vi "camara y sonido.vi"() -> ()   [LabVIEW 2010]
uses:
  <vilib>/sound2/lvsound2.llb/Sound Data Format.ctl
  <vilib>/addons/PixeLINK/Low Level Functions/CAMERA_FEATURES.llb/TDPU-CameraFeatures-PixelFormat.ctl
  <vilib>/sound2/lvsound2.llb/Sound Output Task ID.ctl
  <vilib>/vision/Image Controls.llb/IMAQ Image.ctl
panel:
  in  "Salto a Base":bool
  in  "Comienza Saltos":bool
  out "Estable":bool=TRUE
  out "Saltando":bool=TRUE
  in  "Path":path
  in  "Nombre Imagen":string="foto"
  in  "Numero Ultimo Experimento":i32
  in  "Parametros de Saltos":T1={"Numero de Saltos"=6, "Paso del Salto (Hz)"=100.0, "Tiempo de estabilizacion (s)"=1.0, "Frequencia de estabilizacion (Hz)"=2000.0, "Tiempo de rampa ON (s)"=5.0, "Tiempo de rampa OFF (s)"=1.0}
  in  "Calibrar Sonido":bool
  out "Archivo Actual":path
  out "Guardando Imagen":bool=TRUE
  in  "Compresion":u16(ring)=6 items=["DV Video Encoder", "LogMeIn Video Encoder", "MJPEG Compressor", "Cinepak Codec by Radius", "Intel IYUV codec", "Intel IYUV codec", "Microsoft RLE", "Microsoft Video 1"]
  in  "Nueva Linea?":bool
  in  "Grabar":bool
  in  "Video?":bool
  out "Archivo de texto":path
  out "Selected Path for AVI":path
  out "time (ms)":u32
  out "Contraste":dbl(graph)
  out "Todo Funciona?":bool
  out "Image":T2(plugin-control)
  in  "Tab Control":enum32{"Sound", "Camara"}(tab)
  in  "Sound Controls":T4={"device ID"=0, "sound format"={"sample rate (S/s)"=44000.0, "number of channels"=2, "bits per sample"=16}, "time (ms)"=200.0}
  in  "Sound?":bool
  in  "Frecuencia":dbl
  in  "Selector":u16(ring) items=["776002034"]
  in  "Streeam?":bool
  out "Camara Funciona?":bool
  out "Contraste":dbl
  in  "Camera Parameters":T6 {"Pixel Format" items=["PIXEL_FORMAT_MONO8", "PIXEL_FORMAT_MONO16", "PIXEL_FORMAT_YUV422", "PIXEL_FORMAT_BAYER8_GRBG", "PIXEL_FORMAT_BAYER16_GRBG", "PIXEL_FORMAT_RGB24", "PIXEL_FORMAT_RGB48", "PIXEL_FORMAT_BAYER8_RGGB", "PIXEL_FORMAT_BAYER8_GBRG ", "PIXEL_FORMAT_BAYER8_BGGR ", "PIXEL_FORMAT_BAYER16_RGGB ", "PIXEL_FORMAT_BAYER16_GBRG", "PIXEL_FORMAT_BAYER16_BGGR", "PIXEL_FORMAT_RGB32"]}
  in  "stop":bool
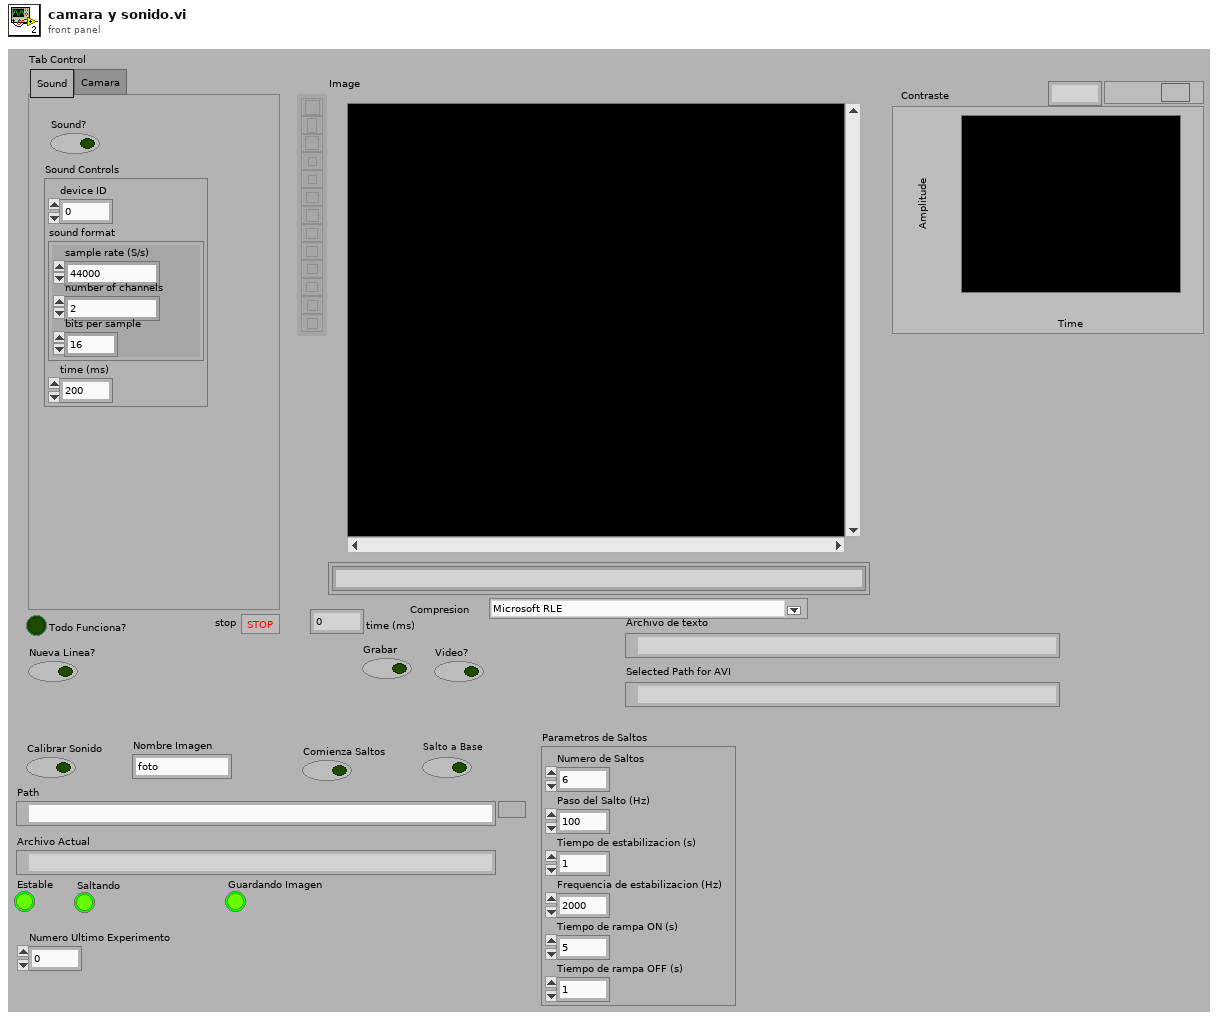
[diagram p1: front panel]
types:
  T1 = cluster{"Numero de Saltos":i32, "Paso del Salto (Hz)":dbl, "Tiempo de estabilizacion (s)":dbl, "Frequencia de estabilizacion (Hz)":dbl, "Tiempo de rampa ON (s)":dbl, "Tiempo de rampa OFF (s)":dbl}
  T2 = typedef "IMAQ Image.ctl" = refnum<image>
  T3 = typedef "Sound Data Format.ctl" = cluster{"sample rate (S/s)":dbl, "number of channels":i32, "bits per sample":i32}
  T4 = cluster{"device ID":u32, "sound format":T3, "time (ms)":dbl}
  T5 = typedef "TDPU-CameraFeatures-PixelFormat.ctl" = u16
  T6 = cluster{"Exposure Time (ms)":dbl, "Gain (dB)":dbl, "Saturation (%)":dbl, "Sharpness (%)":dbl, "Color Temperature":dbl, "ROI":cluster{"Top":i32, "Left":i32, "Width":i32, "Height":i32}, "White Balance Gain (dB)":cluster{"Red":dbl, "Green":dbl, "Blue":dbl}, "Gamma":dbl, "Pixel Format":T5, "FPS (frames/s)":i32}
  T7 = cluster{"hCamera":u32, "Error":errorcluster, "uSerialNumber OUT":u32}
  T8 = typedef "Sound Output Task ID.ctl" = u32
  T9 = cluster{"task ID":T8, "error":errorcluster, "sound format":T3}
  T10 = cluster{"hCamera":u32, "Error":errorcluster, "uSerialNumber":u32}
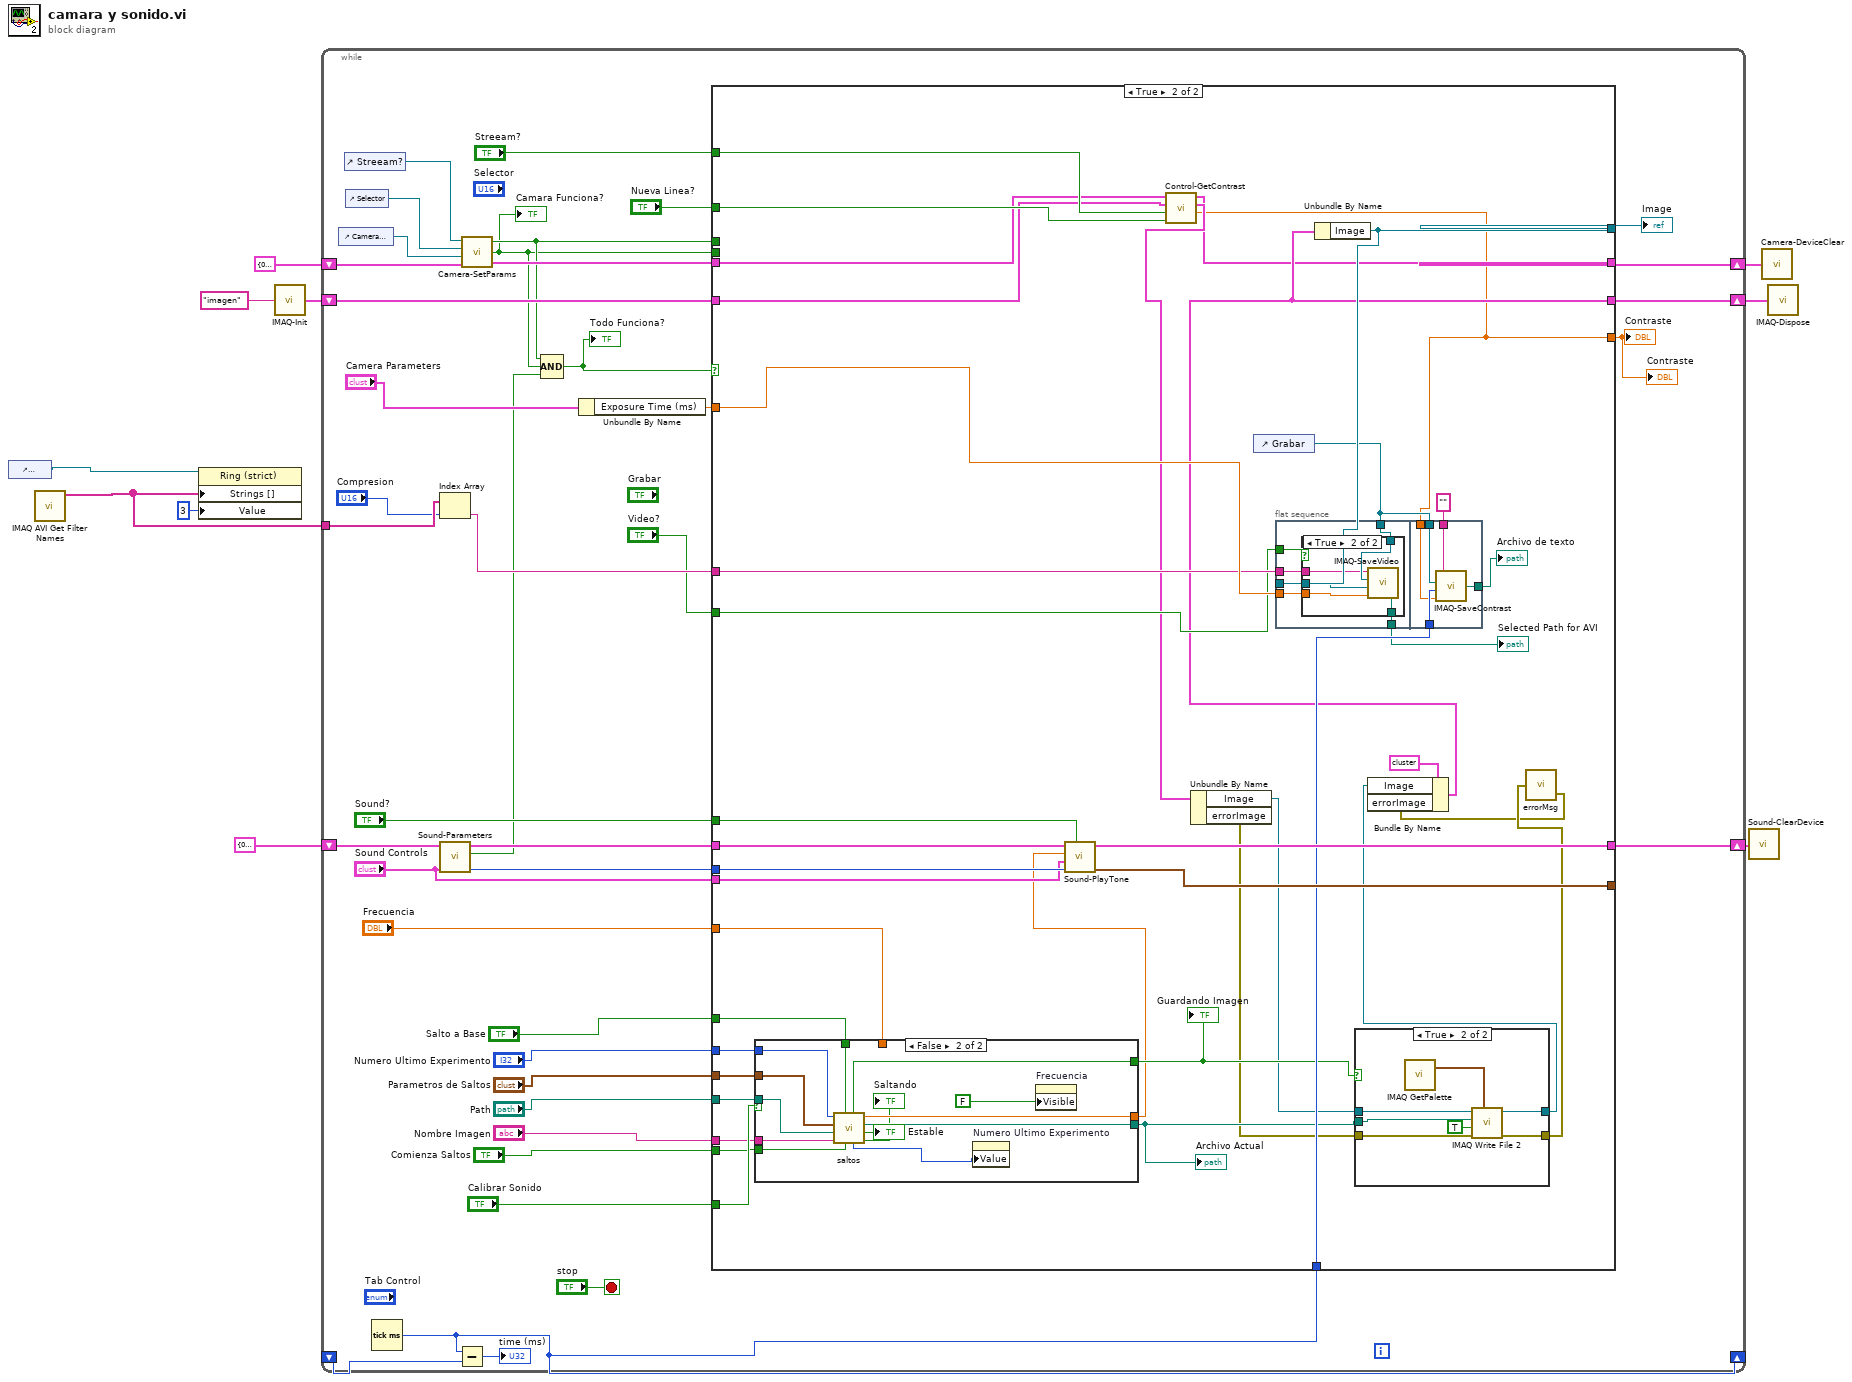
[diagram p0: block diagram]
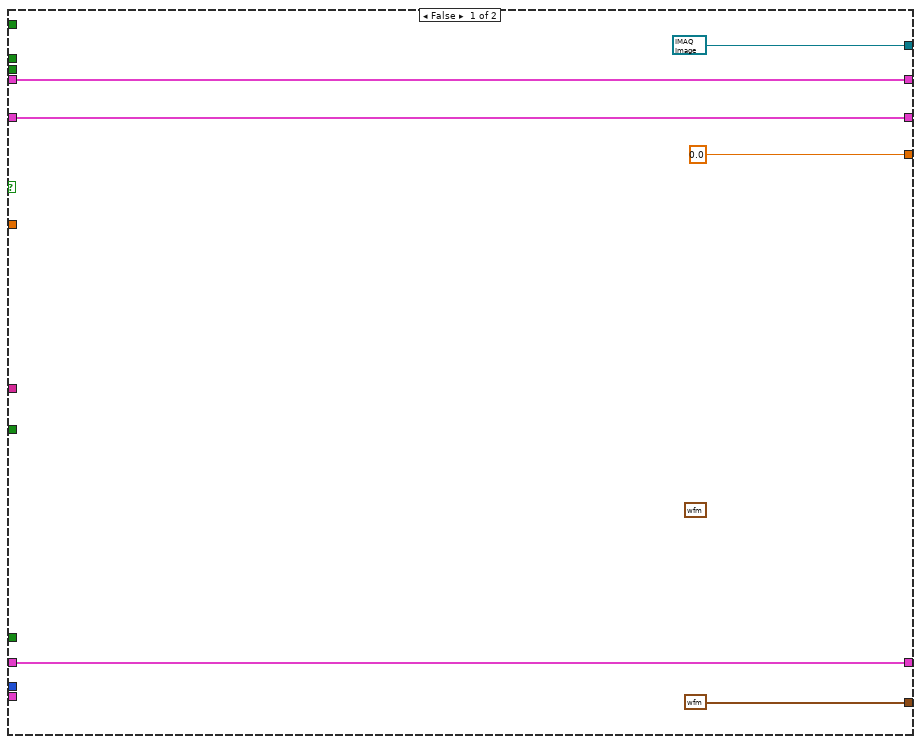
[diagram p2: hidden frame]
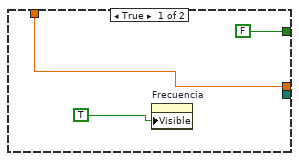
[diagram p4: hidden frame]
diagram:
  n1 = control-ref of="Compresion"() -> (w1:refnum<vi>)
  n2 = call "IMAQ AVI Get Filter Names"() -> ("Filter Names"=w2:string[])  [unwired: 10 in, 1 out]
  n3 = property on="Property Node" class="Ring (strict)"(reference=w1, "Strings []"=w2, "Value"=u16 3) -> ()  [unwired: 1 in, 2 out]
  n4 = call "IMAQ-Init.vi"("Image Name"="imagen") -> ("Image Device OUT"=w7:cluster{"Image":T2, "errorImage":errorcluster})  [unwired: 2 in, 2 out]
  n5 = while {
    shift-right: [w47] -> w9
    shift-left: T9 {"task ID"=0, "error"={"status"=TRUE, "code"=0, "source"=""}, "sound format"={"sample rate (S/s)"=0.0, "number of channels"=0, "bits per sample"=0}} ("Sound Device OUT") -> [w46]
    shift-right: [w35] -> w4
    shift-left: w7 -> [w39]
    shift-right: [w38] -> w5
    shift-left: T7 {"hCamera"=0, "Error"={"status"=FALSE, "code"=0, "source"=""}, "uSerialNumber OUT"=0} ("Camera Device  IN") -> [w37]
    shift-right: [w27] -> _
    shift-left: _ -> [w29]
    tunnel: w2 -> [w26]
    stop <- "stop" stop-if-true
    n6 = control-ref of="Camera Parameters"() -> (w22:refnum<vi>)
    n7 = control-ref of="Streeam?"() -> (w41:refnum<vi>)
    n8 = control-ref of="Selector"() -> (w42:refnum<vi>)
    n9 = Tick Count (ms)() -> (millisecond timer value=w27:u32)
    n10 = Index Array(array=w26, index="Compresion") -> (element=w25:string)
    n11 = call "Sound-Parameters.vi"("Sound Controls"="Sound Controls", "Sound Device IN"=w46) -> ("#samples"=w48:u32, "En funcionamiento?"=w12:bool, "Sound Device OUT"=w49:T9)  [unwired: 3 in]
    n12 = Subtract(x=w27, y=w29) -> (x-y=→"time (ms)":u32)
    n13 = call "Camera-SetParams.vi"("Camera Device  IN"=w37, "Camera Parameters"=w22, "Selector"=w42, "Stream?"=w41) -> ("Camera Device OUT"=w40:T10, "Funciona?"=w31:bool, "Stream? OUT"=w32:bool)
    "Camara Funciona?" <- w31
    n14 = Compound Arithmetic op=AND(w32, w31, w12) -> (w33:bool)
    "Todo Funciona?" <- w33
    n15 = Unbundle By Name("Camera Parameters") -> ("Exposure Time (ms)"=w34:dbl)
    n16 = case shown="True" w33 {
      tunnel: [waveform(dbl) {"t0"=timestamp(0 s since 1904-01-01), "dt"=1.0, "Y"=[]} ("Waveform") w96] -> _
      tunnel: w49 -> [w53 w95]
      tunnel: w48 -> [_ w94]
      tunnel: [w53 w93] -> w47
      tunnel: "Sound?" -> [_ w92]
      tunnel: "Frecuencia" -> [_ w74]
      tunnel: "Sound Controls" -> [_ w91]
      tunnel: w40 -> [w55 w62]
      tunnel: w39 -> [w54 w61]
      tunnel: [w55 w59] -> w38
      tunnel: [T2 refnum ("Image") w90] -> w36
      tunnel: [w54 w67] -> w35
      tunnel: [0.0 ("Contraste") w58] -> w30
      tunnel: w31 -> [_ _]
      tunnel: w32 -> [_ _]
      tunnel: w34 -> [_ w89]
      tunnel: "Streeam?" -> [_ w64]
      tunnel: w27 -> [_ w88]
      tunnel: w25 -> [_ w85]
      tunnel: "Video?" -> [_ w84]
      tunnel: "Nueva Linea?" -> [_ w63]
      tunnel: "Salto a Base" -> [_ w82]
      tunnel: "Numero Ultimo Experimento" -> [_ w81]
      tunnel: "Parametros de Saltos" -> [_ w80]
      tunnel: "Path" -> [_ w79]
      tunnel: "Calibrar Sonido" -> [_ w78]
      tunnel: "Nombre Imagen" -> [_ w77]
      tunnel: "Comienza Saltos" -> [_ w76]
      frame False {
        (unwired) waveform(dbl) {"t0"=timestamp(0 s since 1904-01-01), "dt"=1.0, "Y"=[]} ("Waveform")
      }
      frame True {
        n17 = case shown="False" w78 {
          tunnel: w81 -> [_ w121]
          tunnel: w80 -> [_ w120]
          tunnel: w79 -> [_ w119]
          tunnel: w77 -> [_ w118]
          tunnel: w76 -> [_ w117]
          tunnel: [_ w116] -> w71
          tunnel: [FALSE ("Captura Imagen") w115] -> w75
          tunnel: [w107 w114] -> w73
          tunnel: w82 -> [_ w111]
          tunnel: w74 -> [w107 _]
          frame True {
            n18 = property on="Frecuencia" class="DigNum (strict)"("Visible"=TRUE) -> ()  [unwired: 2 in, 2 out]
          }
          frame False {
            n19 = call "saltos.vi"("Comienza Saltos"=w117, "Secuencial"=w111, "Nombre Imagen"=w118, "Path"=w119, "Parametros de Saltos"=w120, "Numero Ultimo Experimento"=w121) -> ("Tomando Saltos"=→"Saltando":bool, "Estable"=→"Estable":bool, "appended path"=w116:path, "Freq Output"=w114:dbl, "Numero Actual Experimento"=w110:i32, "Captura Imagen"=w115:bool)
            n20 = property on="Numero Ultimo Experimento" class="DigNum (strict)"("Value"=w110) -> ()  [unwired: 2 in, 2 out]
            n21 = property on="Frecuencia" class="DigNum (strict)"("Visible"=FALSE) -> ()  [unwired: 2 in, 2 out]
          }
        }
        "Guardando Imagen" <- w75
        "Archivo Actual" <- w71
        n22 = call "Sound-PlayTone.vi"("sound?"=w92, "# samples"=w94, "Sound Controls"=w91, "Frecuencia"=w73, "Sound Device IN"=w95) -> ("Waveform"=w96:waveform(dbl), "Sound Device OUT"=w93:T9)  [unwired: 3 in]
        n23 = call "Control-GetContrast.vi"("Nueva Linea?"=w63, "Streeam?"=w64, "Image Device IN"=w61, "Camera Device  IN"=w62) -> ("Contraste OUT"=w58:dbl, "Image Device OUT"=w60:cluster{"Image":T2, "errorImage":errorcluster}, "Camera Device OUT"=w59:T7)  [unwired: 1 in]
        n24 = Unbundle By Name(w60) -> ("Image"=w72:T2, "errorImage"=w70:errorcluster)
        n25 = control-ref of="Grabar"() -> (w83:refnum<vi>)
        n26 = flat-sequence {
          tunnel: w83 -> [w127]
          tunnel: w90 -> [w126]
          tunnel: w89 -> [w125]
          tunnel: [w124] -> w87
          tunnel: w85 -> [w123]
          tunnel: w84 -> [w122]
          tunnel: w83 -> [w137]
          tunnel: w88 -> [w136]
          tunnel: w58 -> [w135]
          tunnel: [w134] -> w86
          tunnel: "" ("Status Text") -> [w133]
          frame #0 {
            n27 = case shown="True" w122 {
              tunnel: w127 -> [_ w132]
              tunnel: w126 -> [_ w131]
              tunnel: w125 -> [_ w130]
              tunnel: [_ w129] -> w124
              tunnel: w123 -> [_ w128]
              frame False {
              }
              frame True {
                n28 = call "IMAQ-SaveVideo.vi"("Exposure Time (ms)"=w130, "Image"=w131, "Grabar"=w132, "Compression Filter"=w128) -> ("Selected Path for AVI"=w129:path)
              }
            }
          }
          frame #1 {
            n29 = call "IMAQ-SaveContrast.vi"("contraste"=w135, "tiempo (ms)"=w136, "Grabar"=w137, "Status"=w133) -> ("Archivo de texto"=w134:path)
          }
        }
        n30 = case shown="True" w75 {
          tunnel: w72 -> [w98 w105]
          tunnel: [w98 w104] -> w68
          tunnel: w70 -> [w97 w103]
          tunnel: [w97 w102] -> w66
          tunnel: w71 -> [_ w101]
          frame False {
          }
          frame True {
            n31 = call "IMAQ GetPalette"() -> ("Color Palette"=w100:cluster{"Red":u8, "Green":u8, "Blue":u8}[])  [unwired: 5 in, 1 out]
            n32 = call-poly "IMAQ Write File 2"("Color Palette"=w100, "error in (no error)"=w103, "Compress? (N)"=TRUE, "File Path"=w101, "Image"=w105) -> ("error out"=w102:errorcluster, "Image Out (duplicate)"=w104:T2)  [unwired: 5 in]
          }
        }
        n33 = call "errorMsg.vi"("error IO 2"=w66) -> ("error IO"=w65:errorcluster)  [unwired: 1 out]
        n34 = Bundle By Name(cluster=cluster{"Image":T2, "errorImage":errorcluster} {"Image"=refnum, "errorImage"={"status"=FALSE, "code"=0, "source"=""}} ("Image Device OUT"), "Image"=w68, "errorImage"=w65) -> (w67:cluster{"Image":T2, "errorImage":errorcluster})
        n35 = Unbundle By Name(w67) -> ("Image"=w90:T2)
        "Selected Path for AVI" <- w87
        "Archivo de texto" <- w86
      }
    }
    "Image" <- w36
    "Contraste" <- w30
    "Contraste" <- w30
  }
  n36 = call "Sound-ClearDevice.vi"("Sound Device OUT"=w9) -> ()
  n37 = call "Camera-DeviceClear.vi"("Camera Device OUT"=w5) -> ()
  n38 = call "IMAQ-Dispose.vi"("Image Device IN"=w4) -> ()
